vi "ShooterWheelLogicV3.vi"(0 "Setpoint":dbl, 5 "Process Varaible":dbl, 7 "Feedfoward Voltage":dbl, 9 "SwitchZones":T1, 11 "PID gains":T2, 12 "Error Margin":dbl, 13 "Reset":bool) -> (4 "At Speed":bool, 6 "Motor Output":dbl, 8 "Voltage Output":dbl, 10 "Error":dbl, 15 "Wheel Died":bool)   [LabVIEW 2012]
uses:
  Max'sToolKit/ConvertVoltageToPercentVbs.vi
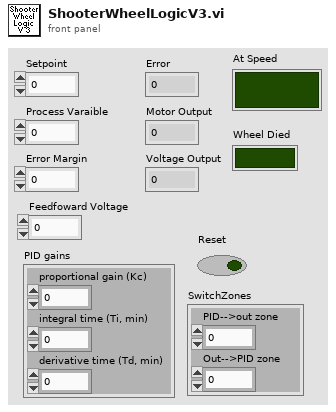
[diagram p1: front panel]
types:
  T1 = cluster{"PID-->out zone":dbl, "Out-->PID zone":dbl}
  T2 = cluster{"proportional gain (Kc)":dbl, "integral time (Ti, min)":dbl, "derivative time (Td, min)":dbl}
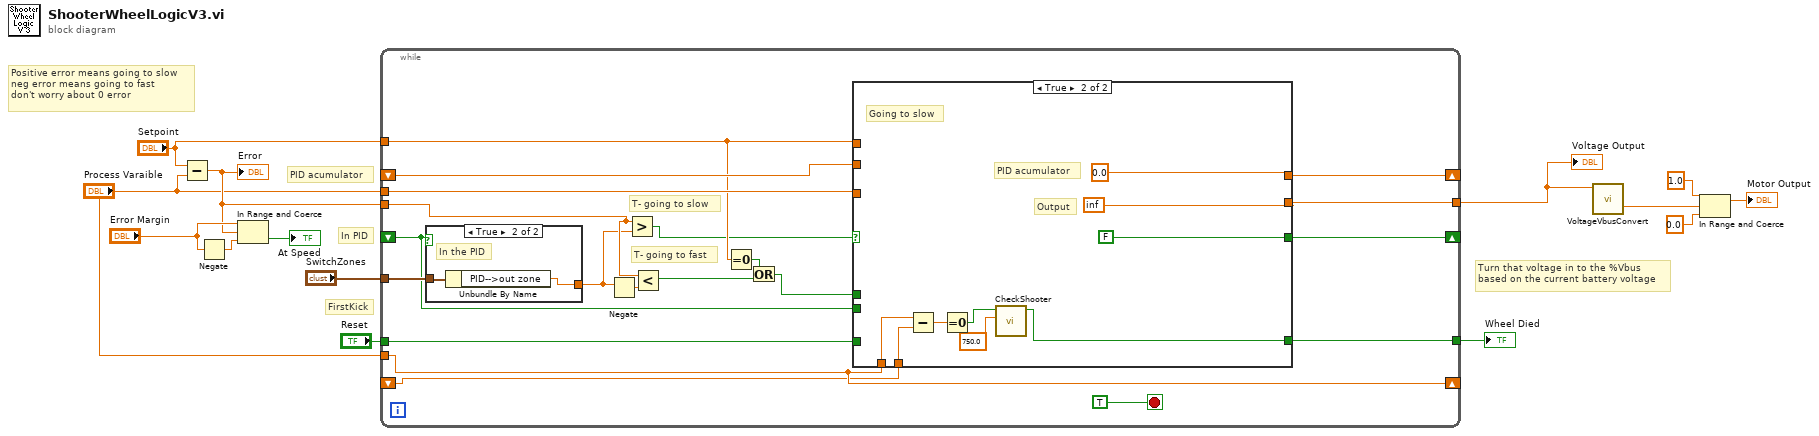
[diagram p0: block diagram]
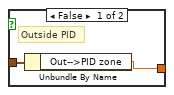
[diagram p2: hidden frame]
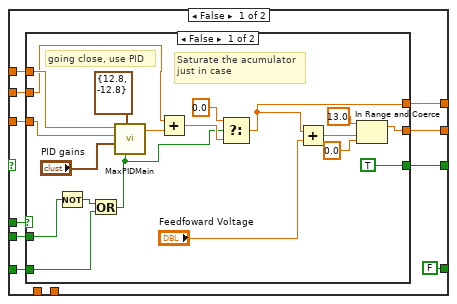
[diagram p3: hidden frame]
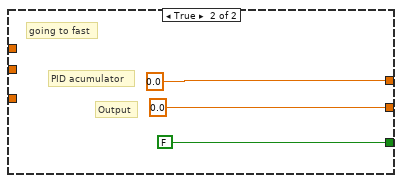
[diagram p4: hidden frame]
diagram:
  # "Turn that voltage in to the %Vbus\nbased on the current battery voltage"
  # "In PID"
  # "PID acumulator"
  # "FirstKick"
  # "Positive error means going to slow\nneg error means going to fast\ndon't worry about 0 error"
  n1 = Subtract(x="Setpoint", y="Process Varaible") -> (x-y=w4:dbl)
  "Error" <- w4
  n2 = Negate(x="Error Margin") -> (-x=w11:dbl)
  n3 = In Range and Coerce(upper limit="Error Margin", x=w4, lower limit=w11) -> (In Range?=→"At Speed":bool)  [unwired: 1 out]
  n4 = while {
    tunnel: "Setpoint" -> [w24]
    tunnel: "Process Varaible" -> [w34]
    tunnel: "Reset" -> [w33]
    shift-right: [w30] -> _
    shift-left: _ -> [w31]
    tunnel: [w29] -> w6
    shift-right: [w28] -> _
    shift-left: _ -> [w15]
    tunnel: w4 -> [w21]
    tunnel: "Process Varaible" -> [w19]
    shift-right: [w19] -> _
    shift-left: _ -> [w18]
    tunnel: "SwitchZones" -> [w17]
    tunnel: [w16] -> w1
    stop <- TRUE stop-if-true
    # "T- going to fast"
    # "T- going to slow"
    n5 = case shown="True" w15 {
      tunnel: [w35 w38] -> w20
      tunnel: w17 -> [w36 w37]
      frame False {
        # "Outside PID"
        n6 = Unbundle By Name(w36) -> ("Out-->PID zone"=w35:dbl)
      }
      frame True {
        # "In the PID"
        n7 = Unbundle By Name(w37) -> ("PID-->out zone"=w38:dbl)
      }
    }
    n8 = Negate(x=w20) -> (-x=w25:dbl)
    n9 = Greater?(x=w21, y=w20) -> (0:w22:bool)
    n10 = Less?(x=w21, y=w25) -> (x < y?=w26:bool)
    n11 = Equal To 0?(x=w24) -> (x = 0?=w27:bool)
    n12 = Or(x=w27, y=w26) -> (x .or. y?=w23:bool)
    n13 = case shown="True" w22 {
      tunnel: w23 -> [w48 _]
      tunnel: w24 -> [w47 _]
      tunnel: w34 -> [w46 _]
      tunnel: w33 -> [w45 _]
      tunnel: w31 -> [w44 _]
      tunnel: [w43 0.0 ("lower limit")] -> w30
      tunnel: [w42 inf] -> w29
      tunnel: [w41 FALSE] -> w28
      tunnel: w19 -> [_ w76]
      tunnel: w18 -> [_ w75]
      tunnel: [FALSE ("Good to shoot") w71] -> w16
      tunnel: w15 -> [w39 _]
      frame False {
        n14 = case shown="False" w48 {
          tunnel: w47 -> [w65 _]
          tunnel: w46 -> [w64 _]
          tunnel: w45 -> [w51 _]
          tunnel: w44 -> [w59 _]
          tunnel: [w55 0.0 ("lower limit")] -> w43
          tunnel: [w53 0.0 ("lower limit")] -> w42
          tunnel: [TRUE FALSE] -> w41
          tunnel: w39 -> [w49 _]
          frame False {
            # "Saturate the acumulator\njust in case"
            # "going close, use PID"
            n15 = Not(x=w49) -> (.not. x?=w50:bool)
            n16 = Or(x=w50, y=w51) -> (x .or. y?=w52:bool)
            n17 = call "MaxPIDMain.vi"("Reset"=w52, "Output Range"=cluster{"output high":dbl, "output low":dbl} {"output high"=12.8, "output low"=-12.8} ("output range"), "PID gains"="PID gains", "process variable"=w64, "setpoint"=w65) -> ("Output"=w62:dbl)  [unwired: 5 in, 1 out]
            n18 = Add(x=w59, y=w62) -> (x+y=w57:dbl)
            n19 = Select(t=0.0 ("lower limit"), s=w52, f=w57) -> (s? t:f=w55:dbl)
            n20 = Add(x=w55, y="Feedfoward Voltage") -> (x+y=w56:dbl)
            n21 = In Range and Coerce(upper limit=13.0, x=w56, lower limit=0.0) -> (coerced(x)=w53:dbl)  [unwired: 1 out]
          }
          frame True {
            # "Output"
            # "PID acumulator"
            # "going to fast"
          }
        }
      }
      frame True {
        # "Output"
        # "PID acumulator"
        # "Going to slow"
        n22 = Subtract(x=w76, y=w75) -> (x-y=w74:dbl)
        n23 = Equal To 0?(x=w74) -> (x = 0?=w73:bool)
        n24 = call "CheckShooter.vi"("Time for happy (ms)"=750.0, "Shooter Good?"=w73) -> ("Good to shoot"=w71:bool)  [unwired: 9 in]
      }
    }
  }
  "Voltage Output" <- w6
  "Wheel Died" <- w1
  n25 = call-poly "VoltageVbusConvert.vi"("Voltage"=w6) -> ("Vbus"=w8:dbl)  [unwired: 10 in]
  n26 = In Range and Coerce(upper limit=1.0, x=w8, lower limit=0.0) -> (coerced(x)=→"Motor Output":dbl)  [unwired: 1 out]
